vi "KickForceTestMeanAndStd.vi"(6 "InitialKickForce2DArray":dbl[][](array[numeric]), 8 "error in (no error)":errorcluster, 9 "firstCall":bool, 10 "ResultKickForce2DArray":dbl[][](array[numeric]), 11 "Game in":refnum<class "Game.lvclass">) -> (0 "error out":errorcluster, 1 "KickForceSTD":dbl[][](array[numeric]), 2 "KickForceMean":dbl[][](array[numeric]), 3 "Game out":refnum<class "Game.lvclass">)   [LabVIEW 2023, in "Game.lvclass"]
uses:
  Game.lvclass
  <vilib>/Analysis/NI_AALBase.lvlib
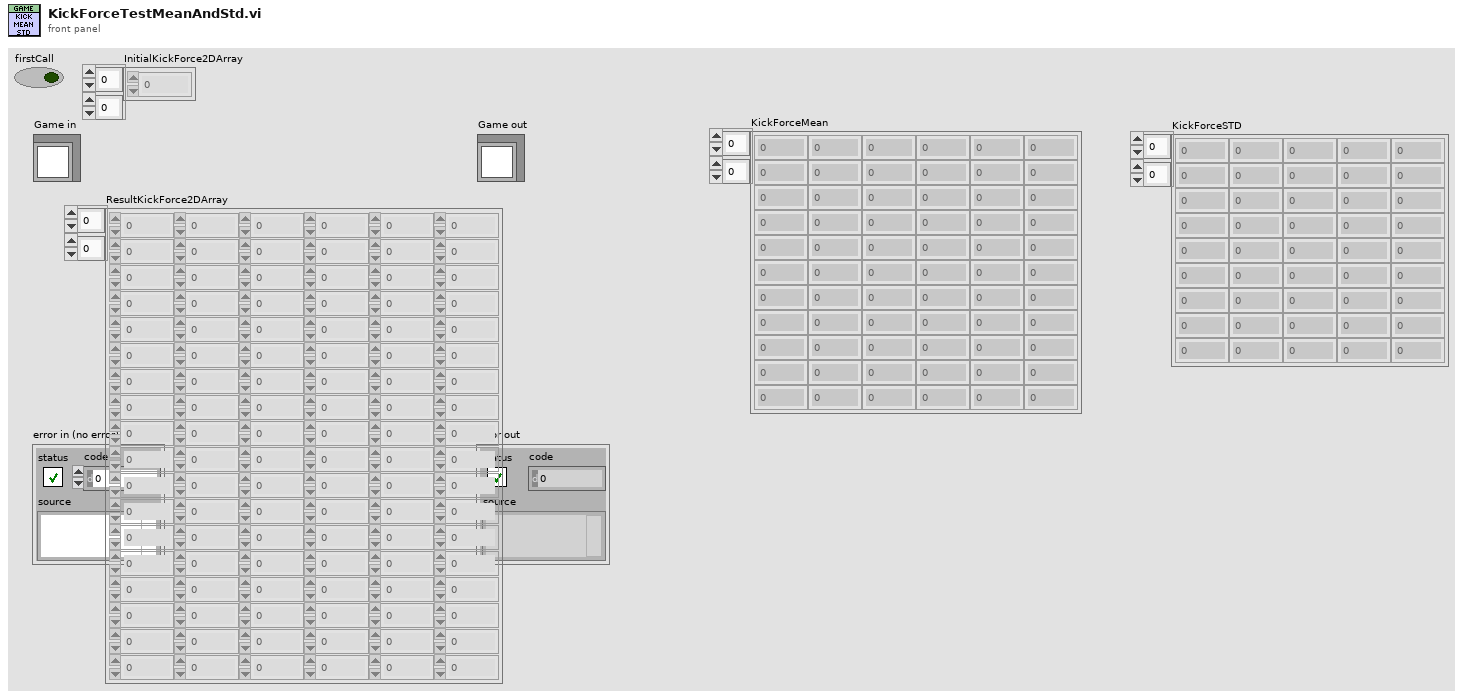
[diagram p1: front panel]
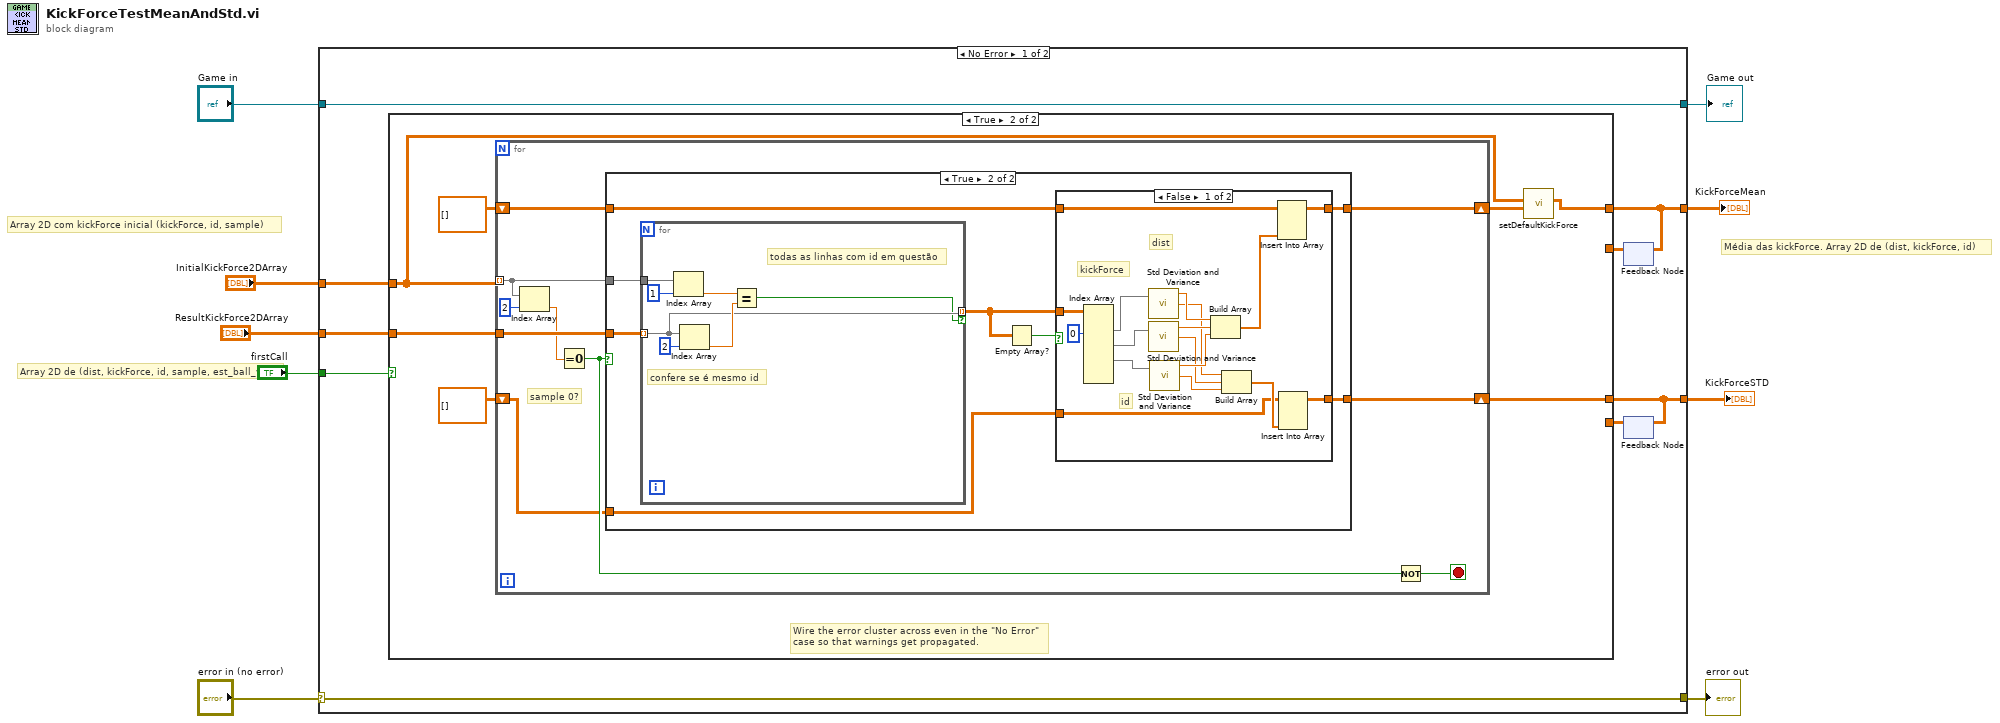
[diagram p0: block diagram]
diagram:
  # "Média das kickForce. Array 2D de (dist, kickForce, id)"
  # "Array 2D com kickForce inicial (kickForce, id, sample)"
  # "Array 2D de (dist, kickForce, id, sample, est_ball_vel)"
  n1 = case shown="No Error" "error in (no error)" {
    selector: "error in (no error)" -> [w17 w75]
    tunnel: [w17 w75] -> w8
    tunnel: [w18 w74] -> w6
    tunnel: "Game in" -> [w18 w74]
    tunnel: "ResultKickForce2DArray" -> [w16 _]
    tunnel: [w15 _] -> w5
    tunnel: [w13 _] -> w4
    tunnel: "firstCall" -> [w10 _]
    tunnel: "InitialKickForce2DArray" -> [w11 _]
    frame No Error {
      n2 = feedback #1() -> (w14:dbl[][])  [unwired: 1 in]
      n3 = feedback #2() -> (w12:dbl[][])  [unwired: 1 in]
      n4 = case shown="True" w10 {
        tunnel: w16 -> [_ w27]
        tunnel: [w20 w22] -> w15
        tunnel: [w19 w24] -> w13
        tunnel: w14 -> [w20 _]
        tunnel: w12 -> [w19 _]
        tunnel: w11 -> [_ w21]
        frame False {
        }
        frame True {
          # "Wire the error cluster across even in the \"No Error\"\ncase so that warnings get propagated."
          n5 = for {
            tunnel: w21 -> [w36] mode=indexing
            tunnel: w27 -> [w37]
            shift-right: [w30] -> w23
            shift-left: dbl[][] [] -> [w31]
            shift-right: [w29] -> w24
            shift-left: dbl[][] [] -> [w28]
            stop <- w32 stop-if-true
            # "sample 0?"
            n6 = Index Array(array=w36, index=2) -> (element=w34:dbl)
            n7 = Equal To 0?(x=w34) -> (x = 0?=w33:bool)
            n8 = case shown="True" w33 {
              tunnel: w37 -> [_ w47]
              tunnel: w36 -> [_ w46]
              tunnel: w31 -> [w39 w45]
              tunnel: [w39 w44] -> w30
              tunnel: [w38 w43] -> w29
              tunnel: w28 -> [w38 w42]
              frame False {
              }
              frame True {
                n9 = for {
                  tunnel: w47 -> [w70] mode=indexing
                  tunnel: w46 -> [w73]
                  tunnel: [w70] -> w41 mode=indexing if=w69
                  # "confere se é mesmo id"
                  # "todas as linhas com id em questão"
                  n10 = Index Array(array=w73, index=1) -> (element=w72:dbl)
                  n11 = Index Array(array=w70, index=2) -> (element=w71:dbl)
                  n12 = Equal?(x=w72, y=w71) -> (x = y?=w69:bool)
                }
                n13 = Empty Array?(array=w41) -> (empty?=w40:bool)
                n14 = case shown="False" w40 {
                  tunnel: w41 -> [w64 _]
                  tunnel: w45 -> [w55 w66]
                  tunnel: [w54 w66] -> w44
                  tunnel: [w49 w65] -> w43
                  tunnel: w42 -> [w48 w65]
                  frame False {
                    # "id"
                    # "kickForce"
                    # "dist"
                    n15 = Index Array(array=w64, index (col) #1=0 ("disabled index (col)")) -> (element #1=w62:dbl[], element #2=w61:dbl[], element #3=w60:dbl[])  [unwired: 7 in, 1 out]
                    n16 = call <vilib>:"Std Deviation and Variance.vi"("X"=w62) -> ("mean"=w59:dbl, "standard deviation"=w53:dbl)  [unwired: 1 in, 1 out]
                    n17 = call <vilib>:"Std Deviation and Variance.vi"("X"=w61) -> ("mean"=w58:dbl, "standard deviation"=w52:dbl)  [unwired: 1 in, 1 out]
                    n18 = call <vilib>:"Std Deviation and Variance.vi"("X"=w60) -> ("mean"=w57:dbl, "standard deviation"=w51:dbl)  [unwired: 1 in, 1 out]
                    n19 = Build Array(w59, w58, w57) -> (w56:dbl[])
                    n20 = Build Array(w53, w52, w51) -> (w50:dbl[])
                    n21 = Insert Into Array(array=w55, new element=w56) -> (w54:dbl[][])  [unwired: 2 in]
                    n22 = Insert Into Array(array=w48, new element=w50) -> (w49:dbl[][])  [unwired: 2 in]
                  }
                  frame True {
                  }
                }
              }
            }
            n23 = Not(x=w33) -> (.not. x?=w32:bool)
          }
          n24 = call "setDefaultKickForce.vi"("KickForceMean"=w23, "InitialKickForce2DArray"=w21) -> ("KickForceMeanWithDefaultKickForce"=w22:dbl[][])  [unwired: 7 in, 2 out]
        }
      }
      n25 = feedback-in #1(w15) -> ()
      n26 = feedback-in #2(w13) -> ()
    }
    frame Error {
    }
  }
  "error out" <- w8
  "Game out" <- w6
  "KickForceMean" <- w5
  "KickForceSTD" <- w4
